vi "CalTest.vi"() -> ()   [LabVIEW 2020]
uses:
  robot code/Subsystems/MySubsystem/MySubsystem_Global.vi
panel:
  in  "Cals/MySubsystem/BoolVariable1":bool
  in  "Cals/MySubsystem/StringVariable1":string
  in  "Cals/MySubsystem/DblVariable3":dbl
  in  "stop":bool
  in  "Cals/MySubsystem/DblVariable2":dbl
  in  "Cals/MySubsystem/DblVariable1":dbl
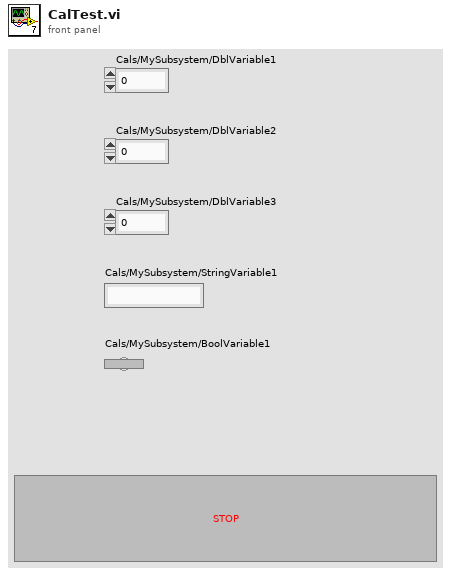
[diagram p1: front panel]
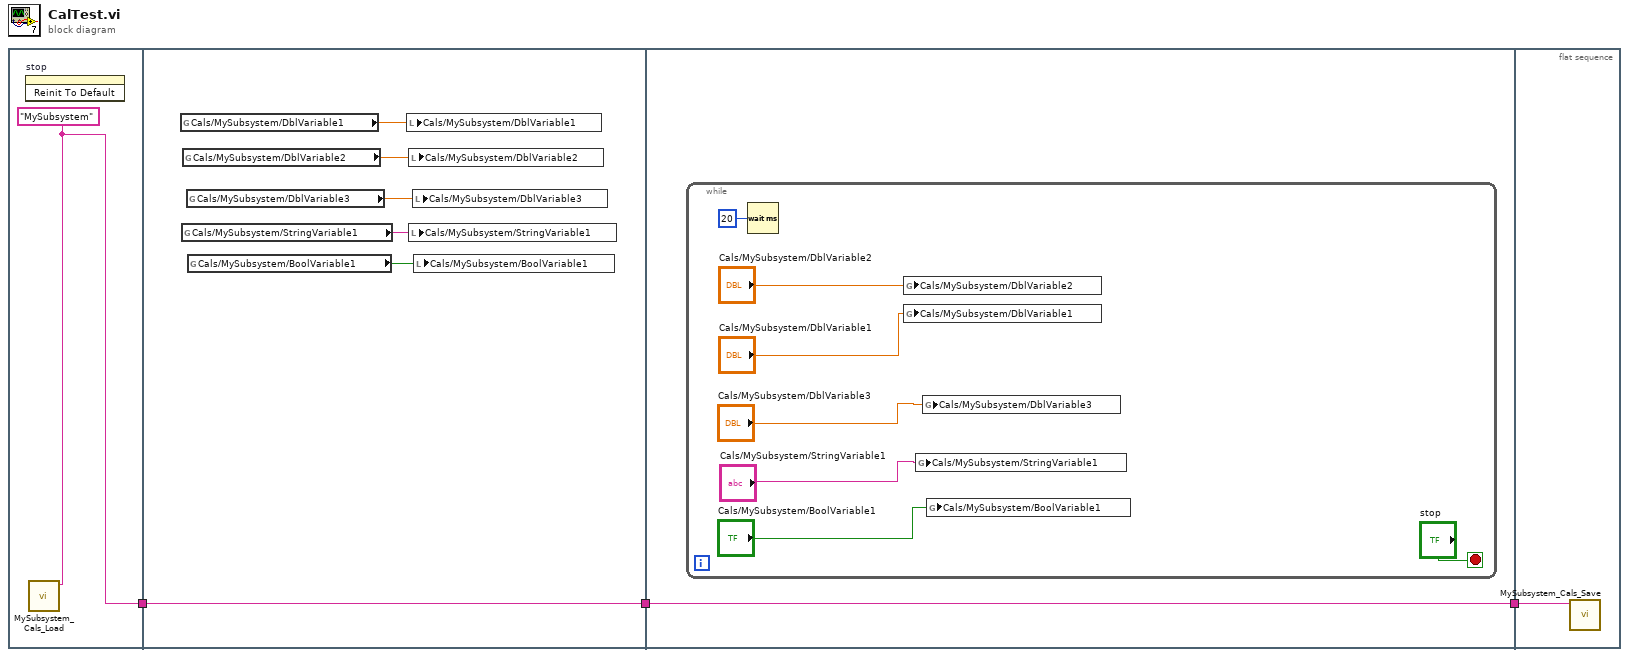
[diagram p0: block diagram]
diagram:
  n1 = flat-sequence {
    tunnel: [w4] -> w2
    tunnel: w2 -> [w10]
    tunnel: [w10] -> w1
    tunnel: [w11] -> w3
    tunnel: w1 -> [w11]
    tunnel: w3 -> [w19]
    frame #0 {
      w4 = "MySubsystem" ("Subsystem")
      n2 = invoke on="stop" class="Bool (strict)" method="Reinit To Default"() -> ()  [unwired: 3 in, 3 out]
      n3 = call "MySubsystem_Cals_Load.vi"("Subsystem"=w4) -> ()  [unwired: 11 in]
    }
    frame #1 {
      n4 = global read "MySubsystem_Global.vi" "Cals/MySubsystem/DblVariable1"() -> (w9:dbl)
      n5 = global read "MySubsystem_Global.vi" "Cals/MySubsystem/StringVariable1"() -> (w6:string)
      n6 = global read "MySubsystem_Global.vi" "Cals/MySubsystem/DblVariable2"() -> (w8:dbl)
      n7 = global read "MySubsystem_Global.vi" "Cals/MySubsystem/DblVariable3"() -> (w7:dbl)
      n8 = global read "MySubsystem_Global.vi" "Cals/MySubsystem/BoolVariable1"() -> (w5:bool)
      n9 = local write "Cals/MySubsystem/DblVariable1"(w9) -> ()
      n10 = local write "Cals/MySubsystem/DblVariable2"(w8) -> ()
      n11 = local write "Cals/MySubsystem/StringVariable1"(w6) -> ()
      n12 = local write "Cals/MySubsystem/DblVariable3"(w7) -> ()
      n13 = local write "Cals/MySubsystem/BoolVariable1"(w5) -> ()
    }
    frame #2 {
      n14 = while {
        stop <- "stop" stop-if-true
        n15 = Wait (ms)(milliseconds to wait=u32 20) -> ()  [unwired: 1 out]
        n16 = global write "MySubsystem_Global.vi" "Cals/MySubsystem/DblVariable2"("Cals/MySubsystem/DblVariable2") -> ()
        n17 = global write "MySubsystem_Global.vi" "Cals/MySubsystem/DblVariable1"("Cals/MySubsystem/DblVariable1") -> ()
        n18 = global write "MySubsystem_Global.vi" "Cals/MySubsystem/StringVariable1"("Cals/MySubsystem/StringVariable1") -> ()
        n19 = global write "MySubsystem_Global.vi" "Cals/MySubsystem/DblVariable3"("Cals/MySubsystem/DblVariable3") -> ()
        n20 = global write "MySubsystem_Global.vi" "Cals/MySubsystem/BoolVariable1"("Cals/MySubsystem/BoolVariable1") -> ()
      }
    }
    frame #3 {
      n21 = call "MySubsystem_Cals_Save.vi"("Subsystem"=w19) -> ()  [unwired: 10 in, 1 out]
    }
  }
